vi "Actor Core.vi"(8 "error in":errorcluster, 11 "Red Pitaya in":refnum<class "Red Pitaya.lvclass">) -> (0 "error out":errorcluster, 3 "Actor out":refnum<class "Actor.lvclass">)   [LabVIEW 2015]
doc: "(<B>Filename</B>: Actor Framework.lvlib:Actor.lvclass:Actor Core.vi)\n\nReceives messages to the actor, reacts to them, and initiates any error handling that may shut the actor down.\n\nDescendant classes may override this VI to append parallel tasks for the actor to complete while it handles messages. Overrides use the Call Parent Method node."
uses:
  Mag Lab Measure/Mag Lab Root/Mag Lab Root.lvclass
  Mag Lab Measure/Mag Lab Root Messages/Arm Msg/Arm Msg.lvclass
  <vilib>/ActorFramework/Actor/Actor.lvclass
  Red Pitaya.lvclass
panel:
  in  "Arm":bool
  out "Trigger state":bool
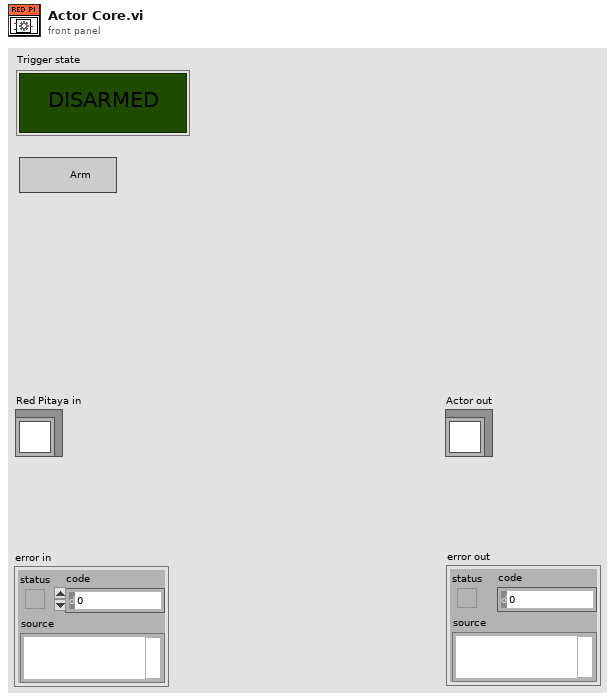
[diagram p1: front panel]
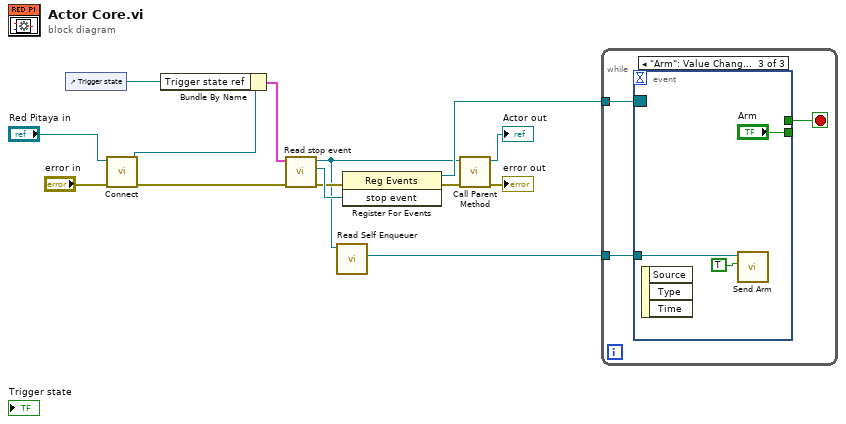
[diagram p0: block diagram]
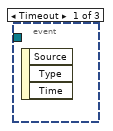
[diagram p2: hidden frame]
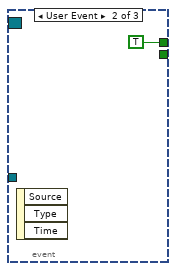
[diagram p3: hidden frame]
diagram:
  n1 = control-ref of="Trigger state"() -> (w6:refnum<vi>)
  n2 = call "Connect.vi"("error in (no error)"="error in", "Red Pitaya in"="Red Pitaya in") -> ("error out"=w1:errorcluster, "Red Pitaya out"=w3:refnum<class "Red Pitaya.lvclass">)  [unwired: 8 in]
  n3 = Bundle By Name(cluster=w3, "Trigger state ref"=w6) -> (w7:cluster{})
  n4 = call "Read stop event.vi"("error in (no error)"=w1, "Mag Lab Root in"=w7) -> ("error out"=w10:errorcluster, "stop event"=w11:refnum<user-event>, "Mag Lab Root out"=w5:refnum<class "Mag Lab Root.lvclass">)  [unwired: 7 in]
  n5 = call <vilib>:"Read Self Enqueuer.vi"("Actor"=w5) -> ("Self Enqueuer"=w4:refnum<class "Message Enqueuer.lvclass">)  [unwired: 10 in]
  n6 = register-events(error in=w10, w11) -> (reference out=w8:refnum<event-registration>, error out=w9:errorcluster)  [unwired: 1 in]
  n7 = call-parent "Call Parent Method"("error in"=w9, "Mag Lab Measure Base in"=w5) -> ("error out"=→"error out":errorcluster, "Actor out"=→"Actor out":refnum<class "Actor.lvclass">)  [unwired: 8 in]
  n8 = while {
    tunnel: w8 -> [w17]
    tunnel: w4 -> [w15]
    stop <- w16 stop-if-true
    n9 = event shown="[2] \"Arm\": Value Change" {
      selector: w17 -> [_ _ _]
      dyn-events: _ -> [_ _ _]
      timeout: _ -> [_ _ _]
      tunnel: [_ TRUE _] -> w16
      tunnel: [_ _ "Arm"] -> _
      tunnel: w15 -> [_ _ w20]
      event Timeout {
        n10 = event-data() -> ()  [unwired: 1 in, 3 out]
      }
      event User Event {
        n11 = event-data() -> ()  [unwired: 1 in, 3 out]
      }
      event "Arm": Value Change {
        n12 = event-data() -> ()  [unwired: 1 in, 3 out]
        n13 = call "Send Arm.vi"("Arm"=TRUE, "Message Enqueuer"=w20) -> ()  [unwired: 8 in, 2 out]
      }
    }
  }
